vi "Teleop.vi"(10 "Match Info":T1={"Autonomous Elapsed Seconds"=0.0, "TeleOp Elapsed Seconds"=0.0, "Disabled Elapsed Seconds"=0.0, "Visited Autonomous"=FALSE, "Visited TeleOp"=FALSE, "Visited Disabled"=FALSE, "Autonomous Settings"={"Autonomous Style"=enum."Independent", "VI Refnum"=refnum}}, 11 "Call Context":T2) -> ()   [LabVIEW 2020]
doc: "This VI is called for each TeleOp packet received from the DS where the robot is not disabled. It is often used to read from the joysticks and update I/O or to update setpoints for timed control loops. It should complete and return within 20 milliseconds or it may miss DS packets."
uses:
  <vilib>/Rock Robotics/WPI/DriverStation/WPI_DriverStationDerivedRobotMode.ctl
  <vilib>/Rock Robotics/WPI/DriverStation/WPI_DriverStationMatch Info.ctl
  <vilib>/Rock Robotics/WPI/ThirdParty/Phoenix-LabVIEW/Motor Controller/Controls/CTRE_Phoenix_MotorControl_ControlMode.ctl
  <vilib>/Rock Robotics/WPI/Utilities/WPI_GetSetVariantRefNum.vi
  <vilib>/Rock Robotics/WPI/ThirdParty/Phoenix-LabVIEW/Motor Controller/Get/CTRE_Phoenix_MotorController_GetSelectedSensorData.vi
panel:
  out "Steering BL Position":i32
  out "Steering BR Position":i32
  out "Steering FL Position":i32
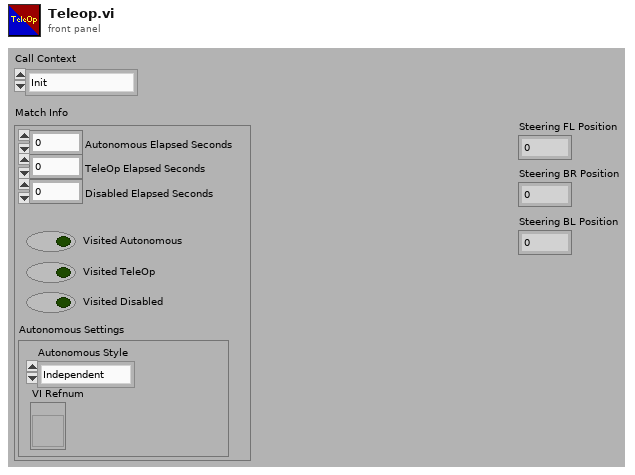
[diagram p1: front panel]
types:
  T1 = typedef "WPI_DriverStationMatch Info.ctl" = cluster{"Autonomous Elapsed Seconds":dbl, "TeleOp Elapsed Seconds":dbl, "Disabled Elapsed Seconds":dbl, "Visited Autonomous":bool, "Visited TeleOp":bool, "Visited Disabled":bool, "Autonomous Settings":cluster{"Autonomous Style":enum16{"Iterative", "Independent"}, "VI Refnum":refnum<vi>}}
  T2 = typedef "WPI_DriverStationDerivedRobotMode.ctl" = enum16{"Init", "Execute", "Stop"}
  T3 = typedef "CTRE_Phoenix_MotorControl_ControlMode.ctl" = u16
  T4 = typedef "WPI_MotorControlDeviceRef.ctl" = cluster{"DeviceStatus":errorcluster, "Type":T5, "PWM":cluster{"PWM Channel":T6, "DeadBand":T7}, "CAN":cluster{"Device Number":u8, "SetOutput VI Ref":variant, "GetOutput VI Ref":variant, "Enable VI Ref":variant, "Disable VI Ref":variant, "Data":variant}, "Invert":bool, "DIO PWM":cluster{"PWM \"Enable\" Channel":T6, "DIOChannel":T8, "PWM Rate":dbl}}
  T5 = typedef "WPI_MotorControlType.ctl" = enum16{"PWM", "CAN", "DIO PWM"}
  T6 = typedef "FPGA_DIOPWMChannel.ctl" = enum8{"PWM 0", "PWM 1", "PWM 2", "PWM 3", "PWM 4", "PWM 5", "PWM 6", "PWM 7", "PWM 8", "PWM 9", "PWM MXP 0", "PWM MXP 1", "PWM MXP 2", "PWM MXP 3", "PWM MXP 4", "PWM MXP 5", "PWM MXP 6", "PWM MXP 7", "PWM MXP 8", "PWM MXP 9", "Invalid"}
  T7 = typedef "WPI_PWMDeadband.ctl" = cluster{"Name":string, "maxPositivePwm":i32, "minPositivePwm":i32, "centerPwm":i32, "maxNegativePwm":i32, "minNegativePwm":i32, "angularRange":u16}
  T8 = typedef "FPGA_DIOChannel.ctl" = enum8{"DIO 0", "DIO 1", "DIO 2", "DIO 3", "DIO 4", "DIO 5", "DIO 6", "DIO 7", "DIO 8", "DIO 9", "DIO MXP 0", "DIO MXP 1", "DIO MXP 2", "DIO MXP 3", "DIO MXP 4", "DIO MXP 5", "DIO MXP 6", "DIO MXP 7", "DIO MXP 8", "DIO MXP 9", "DIO MXP 10", "DIO MXP 11", "DIO MXP 12", "DIO MXP 13", "DIO MXP 14", "DIO MXP 15", "SPI Port CS1", "SPI Port CS2", "SPI Port CS3", "SPI Port MISO", "SPI Port MOSI", "Invalid"}
  T9 = typedef "WPI_JoystickDevRef.ctl" = cluster{"Device":T10}
  T10 = typedef "WPI_JoystickDeviceEnum.ctl" = enum16{"USB 0", "USB 1", "USB 2", "USB 3", "USB 4", "USB 5"}
  T11 = cluster{"Yaw":dbl, "Roll":dbl, "Pitch":dbl, "Heading":dbl, "Fused Heading":dbl}
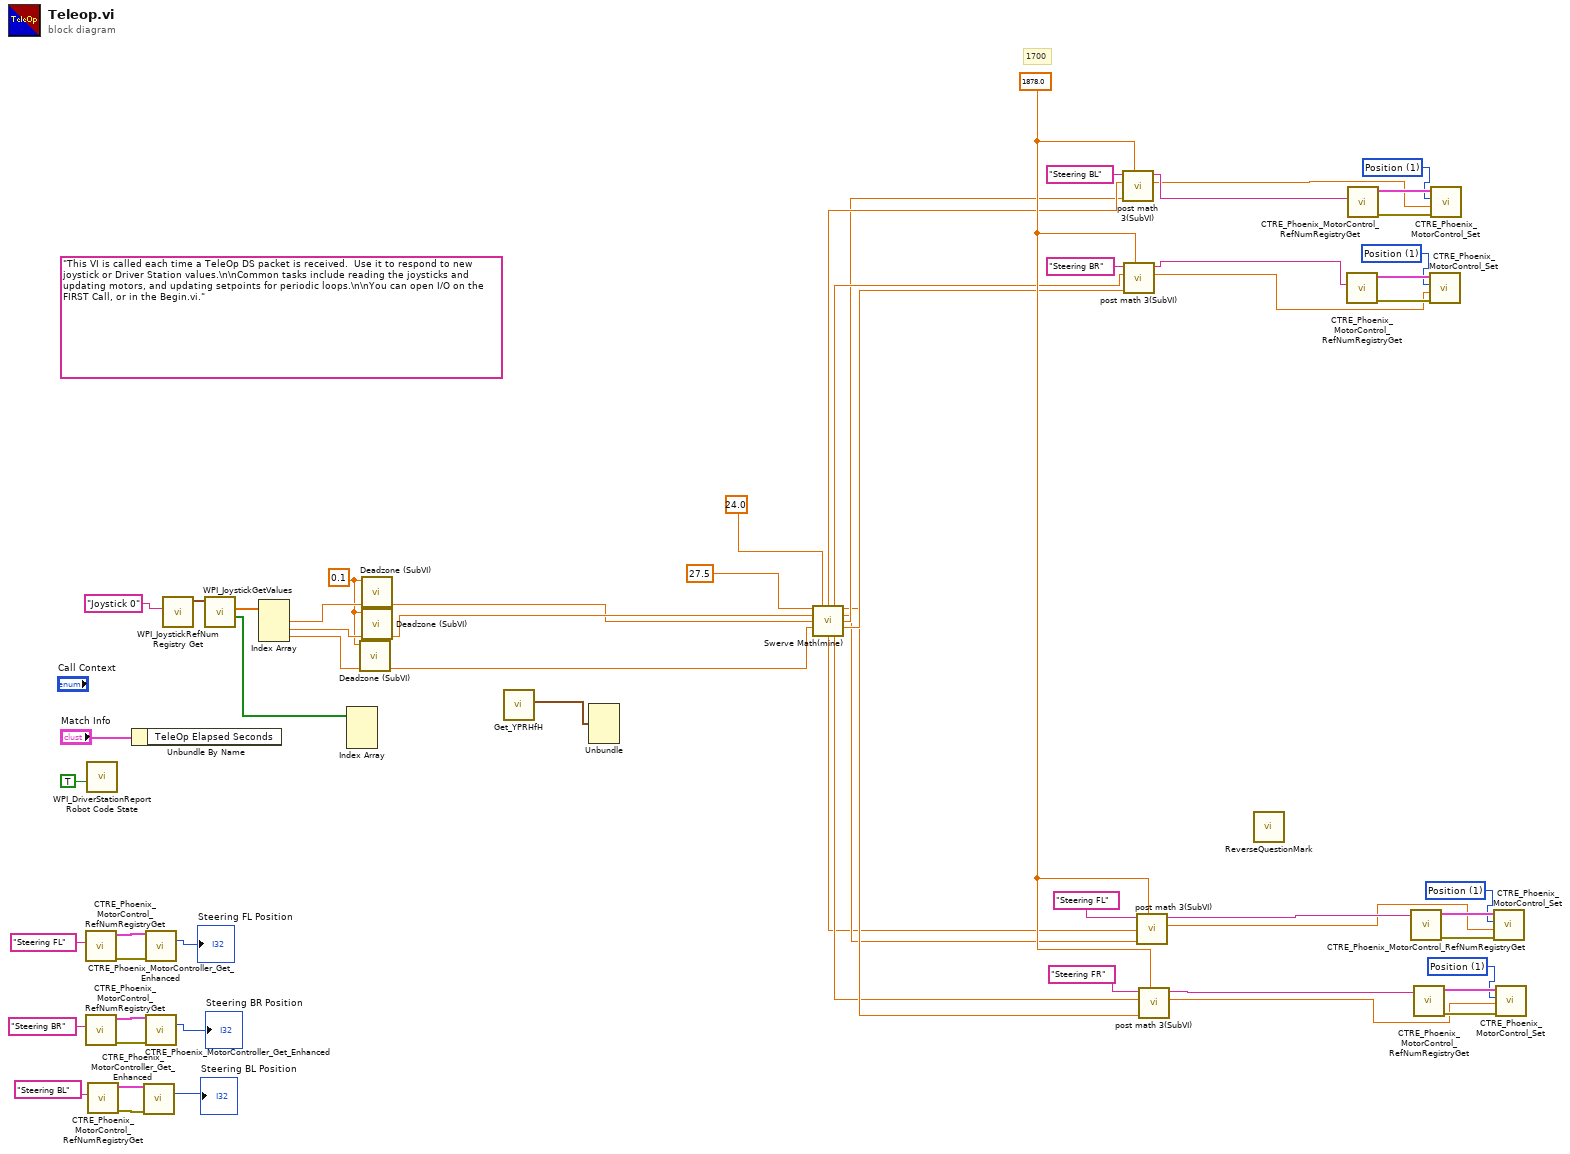
[diagram p0: block diagram]
diagram:
  w19 = T3 1 items=["PercentOutput"=0, "Position"=1, "Velocity"=2, "Current"=3, "Follower"=5, "MotionProfile"=6, "MotionMagic"=7, "MotionProfileArc"=10, "Disabled"=15] ("Control Mode")
  w22 = T3 1 items=["PercentOutput"=0, "Position"=1, "Velocity"=2, "Current"=3, "Follower"=5, "MotionProfile"=6, "MotionMagic"=7, "MotionProfileArc"=10, "Disabled"=15] ("Control Mode")
  w25 = T3 1 items=["PercentOutput"=0, "Position"=1, "Velocity"=2, "Current"=3, "Follower"=5, "MotionProfile"=6, "MotionMagic"=7, "MotionProfileArc"=10, "Disabled"=15] ("Control Mode")
  w30 = T3 1 items=["PercentOutput"=0, "Position"=1, "Velocity"=2, "Current"=3, "Follower"=5, "MotionProfile"=6, "MotionMagic"=7, "MotionProfileArc"=10, "Disabled"=15] ("Control Mode")
  w15 = 1878.0 ("ticks in rotation")
  w53 = 0.1 ("Deadzone")
  (unwired) "This VI is called each time a TeleOp DS packet is received.  Use it to respond to new joystick or Driver Station values.\n\nCommon tasks include reading the joysticks and updating motors, and updating setpoints for periodic loops.\n\nYou can open I/O on the FIRST Call, or in the Begin.vi."
  # "1700"
  n1 = call <vilib>:"CTRE_Phoenix_MotorControl_RefNumRegistryGet.vi"("refnum name"="Steering FL") -> ("error out"=w51:errorcluster, "PhoenixMotorControlDevRef"=w52:T4)  [unwired: 9 in]
  n2 = call <vilib>:"CTRE_Phoenix_MotorControl_RefNumRegistryGet.vi"("refnum name"="Steering BR") -> ("error out"=w47:errorcluster, "PhoenixMotorControlDevRef"=w48:T4)  [unwired: 9 in]
  n3 = call <vilib>:"WPI_DriverStationReport Robot Code State.vi"("TeleOp"=TRUE ("Autonomous")) -> ()  [unwired: 10 in, 1 out]
  n4 = call <vilib>:"CTRE_Phoenix_MotorControl_RefNumRegistryGet.vi"("refnum name"="Steering BL") -> ("error out"=w43:errorcluster, "PhoenixMotorControlDevRef"=w44:T4)  [unwired: 9 in]
  n5 = Unbundle By Name("Match Info") -> ()  [unwired: 1 out]
  n6 = call-poly <vilib>:"CTRE_Phoenix_MotorController_Get_Enhanced.vi"("PhoenixMotorControlDevRef"=w44, "error in"=w43) -> ("Position (Raw Sensor Units)"=→"Steering BL Position":i32)  [unwired: 10 in, 3 out]
  n7 = call-poly <vilib>:"CTRE_Phoenix_MotorController_Get_Enhanced.vi"("PhoenixMotorControlDevRef"=w52, "error in"=w51) -> ("Position (Raw Sensor Units)"=→"Steering FL Position":i32)  [unwired: 10 in, 3 out]
  n8 = call-poly <vilib>:"CTRE_Phoenix_MotorController_Get_Enhanced.vi"("PhoenixMotorControlDevRef"=w48, "error in"=w47) -> ("Position (Raw Sensor Units)"=→"Steering BR Position":i32)  [unwired: 10 in, 3 out]
  n9 = call <vilib>:"WPI_JoystickRefNum Registry Get.vi"("refnum name"="Joystick 0") -> ("JoystickDevRef"=w59:T9)  [unwired: 1 in, 9 out]
  n10 = call <vilib>:"WPI_JoystickGetValues.vi"("JoystickDevRef"=w59) -> ("Buttons"=w40:bool[], "Axes"=w57:dbl[])  [unwired: 6 in, 3 out]
  n11 = Index Array(array=w57) -> (element #1=w56:dbl, element #2=w55:dbl, element #3=w54:dbl)  [unwired: 3 in]
  n12 = Index Array(array=w40) -> ()  [unwired: 3 in, 3 out]
  n13 = call "Deadzone (SubVI).vi"("Input"=w54, "Deadzone"=w53) -> ("Input 2"=w34:dbl)  [unwired: 9 in]
  n14 = call "Deadzone (SubVI).vi"("Input"=w56, "Deadzone"=w53) -> ("Input 2"=w35:dbl)  [unwired: 9 in]
  n15 = call "Deadzone (SubVI).vi"("Input"=w55, "Deadzone"=w53) -> ("Input 2"=w36:dbl)  [unwired: 9 in]
  n16 = call <vilib>:"Get_YPRHfH.vi"() -> ("YRPHfH"=w37:T11)  [unwired: 11 in]
  n17 = Unbundle(w37) -> ()  [unwired: 5 out]
  n18 = call "Swerve Math(mine).vi"("Trackwidth (W)"=27.5, "Wheelbase (L)"=24.0, "Y"=w36, "X"=w35, "Z"=w34) -> ("BL Angle"=w8:dbl, "BR Angle"=w7:dbl, "FR Speed"=w4:dbl, "FL Speed"=w3:dbl, "BL Speed"=w6:dbl, "BR Speed"=w5:dbl, "FL Angle"=w1:dbl, "FR Angle"=w2:dbl)  [unwired: 3 in]
  n19 = call "post math 3(SubVI).vi"("ticks in rotation"=w15, "Motor speed"=w6, "wanted"=w8, "refnum name"="Steering BL") -> ("new position"=w11:dbl, "refnum name 2"=w12:string)  [unwired: 5 in, 1 out]
  n20 = call "post math 3(SubVI).vi"("ticks in rotation"=w15, "Motor speed"=w5, "wanted"=w7, "refnum name"="Steering BR") -> ("new position"=w9:dbl, "refnum name 2"=w10:string)  [unwired: 5 in, 1 out]
  n21 = call "post math 3(SubVI).vi"("ticks in rotation"=w15, "Motor speed"=w3, "wanted"=w1, "refnum name"="Steering FL") -> ("new position"=w28:dbl, "refnum name 2"=w29:string)  [unwired: 5 in, 1 out]
  n22 = call "post math 3(SubVI).vi"("ticks in rotation"=w15, "Motor speed"=w4, "wanted"=w2, "refnum name"="Steering FR") -> ("new position"=w17:dbl, "refnum name 2"=w18:string)  [unwired: 5 in, 1 out]
  n23 = call "ReverseQuestionMark.vi"() -> ()  [unwired: 9 in, 3 out]
  n24 = call <vilib>:"CTRE_Phoenix_MotorControl_RefNumRegistryGet.vi"("refnum name"=w10) -> ("error out"=w20:errorcluster, "PhoenixMotorControlDevRef"=w21:T4)  [unwired: 9 in]
  n25 = call <vilib>:"CTRE_Phoenix_MotorControl_RefNumRegistryGet.vi"("refnum name"=w12) -> ("error out"=w23:errorcluster, "PhoenixMotorControlDevRef"=w24:T4)  [unwired: 9 in]
  n26 = call <vilib>:"CTRE_Phoenix_MotorControl_RefNumRegistryGet.vi"("refnum name"=w29) -> ("error out"=w31:errorcluster, "PhoenixMotorControlDevRef"=w32:T4)  [unwired: 9 in]
  n27 = call <vilib>:"CTRE_Phoenix_MotorControl_RefNumRegistryGet.vi"("refnum name"=w18) -> ("error out"=w26:errorcluster, "PhoenixMotorControlDevRef"=w27:T4)  [unwired: 9 in]
  n28 = call <vilib>:"CTRE_Phoenix_MotorControl_Set.vi"("error in (no error)"=w20, "Output"=w9, "Control Mode"=w19, "PhoenixMotorControlDevRef"=w21) -> ()  [unwired: 6 in, 2 out]
  n29 = call <vilib>:"CTRE_Phoenix_MotorControl_Set.vi"("error in (no error)"=w23, "Output"=w11, "Control Mode"=w22, "PhoenixMotorControlDevRef"=w24) -> ()  [unwired: 6 in, 2 out]
  n30 = call <vilib>:"CTRE_Phoenix_MotorControl_Set.vi"("error in (no error)"=w31, "Output"=w28, "Control Mode"=w30, "PhoenixMotorControlDevRef"=w32) -> ()  [unwired: 6 in, 2 out]
  n31 = call <vilib>:"CTRE_Phoenix_MotorControl_Set.vi"("error in (no error)"=w26, "Output"=w17, "Control Mode"=w25, "PhoenixMotorControlDevRef"=w27) -> ()  [unwired: 6 in, 2 out]
